vi "HR_Zones_Format_Levels.vi"(8 "error in (no error)":errorcluster, 11 "HR Data Structure":T1) -> (0 "error out":errorcluster, 3 "HR Data Structure 2":T1)   [LabVIEW 2021]
uses:
  HR Data Structure.ctl
  Runner's Data.ctl
  Raw Data.ctl
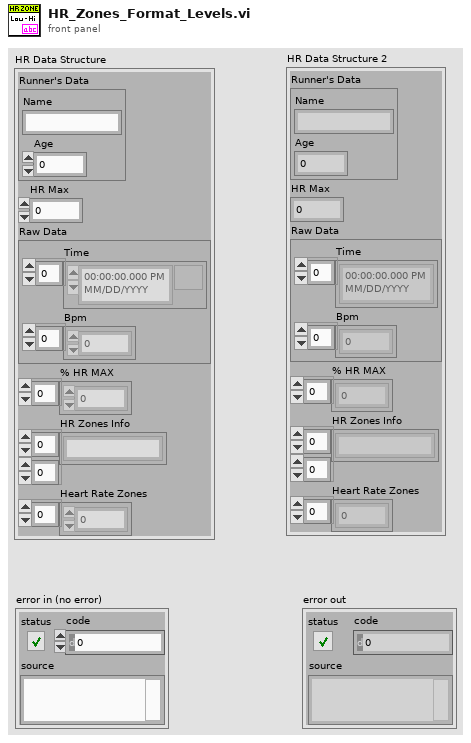
[diagram p1: front panel]
types:
  T1 = typedef "HR Data Structure.ctl" = cluster{"Runner's Data":T2, "HR Max":i32, "Raw Data":T3, "% HR MAX ":dbl[], "HR Zones Info":string[][], "Heart Rate Zones":dbl[]}
  T2 = typedef "Runner's Data.ctl" = cluster{"Name":string, "Age":i32}
  T3 = typedef "Raw Data.ctl" = cluster{"Time":timestamp[], "Bpm":i32[]}
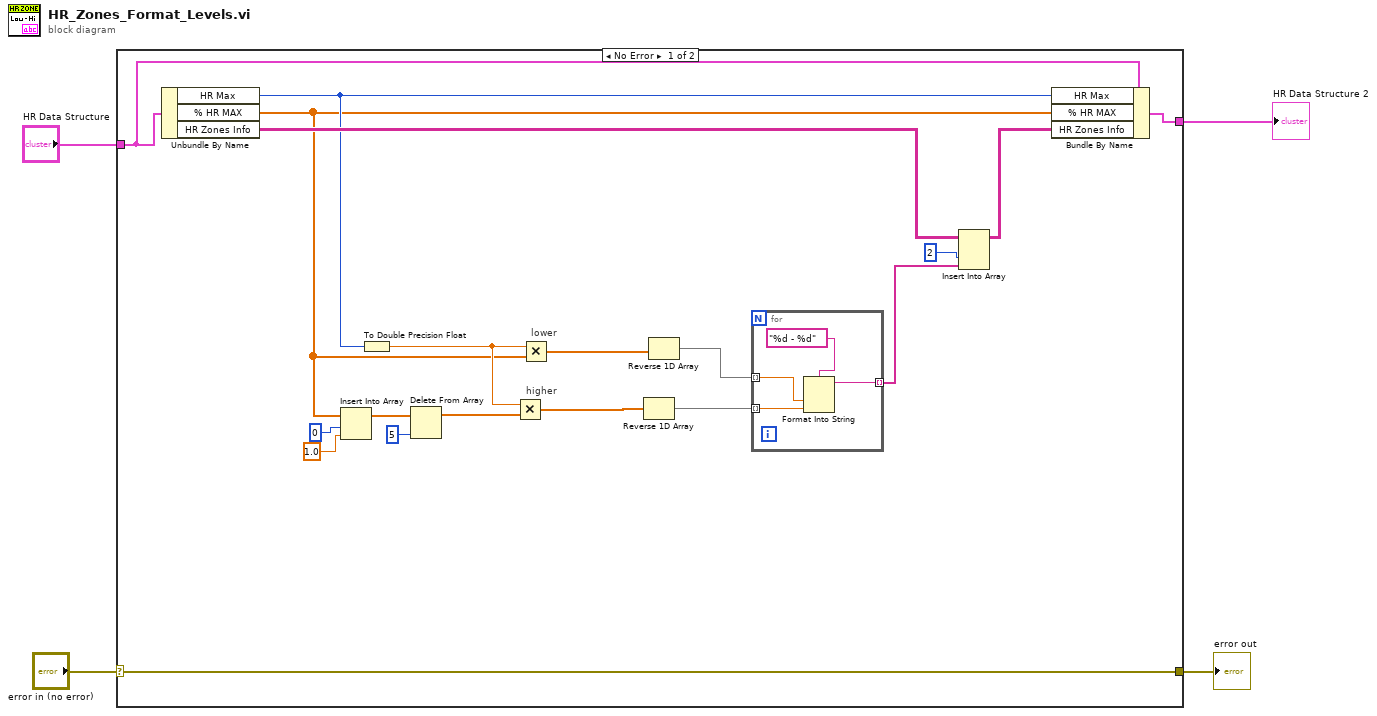
[diagram p0: block diagram]
diagram:
  n1 = case shown="No Error" "error in (no error)" {
    selector: "error in (no error)" -> [w10 w29]
    tunnel: "HR Data Structure" -> [w9 w28]
    tunnel: [w10 w29] -> w2
    tunnel: [w7 w28] -> w1
    frame No Error {
      # "higher"
      # "lower"
      n2 = Unbundle By Name(w9) -> ("HR Max"=w6:i32, "% HR MAX"=w5:dbl[], "HR Zones Info"=w23:string[][])
      n3 = Insert Into Array(array=w5, index=0, new element=1.0) -> (w13:dbl[])
      n4 = To Double Precision Float(number=w6) -> (double precision float=w20:dbl)
      n5 = Delete From Array(array=w13, index=5) -> (array with subset deleted=w16:dbl[])  [unwired: 1 in, 1 out]
      n6 = Multiply(x=w20, y=w16) -> (x*y=w18:dbl[])
      n7 = Multiply(x=w20, y=w5) -> (x*y=w19:dbl[])
      n8 = Reverse 1D Array(array=w18) -> (reversed array=w17:dbl[])
      n9 = Reverse 1D Array(array=w19) -> (reversed array=w15:dbl[])
      n10 = for {
        tunnel: w15 -> [w27] mode=indexing
        tunnel: [w25] -> w22 mode=indexing
        tunnel: w17 -> [w24] mode=indexing
        n11 = Format Into String(format string="%d - %d", w27, w24) -> (resulting string=w25:string)  [unwired: 2 in, 1 out]
      }
      n12 = Insert Into Array(array=w23, index (col)=2, new element=w22) -> (w8:string[][])  [unwired: 1 in]
      n13 = Bundle By Name(cluster=w9, "HR Max"=w6, "% HR MAX"=w5, "HR Zones Info"=w8) -> (w7:T1)
    }
    frame Error {
    }
  }
  "error out" <- w2
  "HR Data Structure 2" <- w1
